vi "Read next.vi"(8 "error in (no error)":errorcluster, 11 "NodeType in":refnum<class "ListNodeVirtual.lvclass">) -> (0 "error out":errorcluster, 2 "next":refnum<data-value>, 3 "NodeType out":refnum<class "ListNodeVirtual.lvclass">)   [LabVIEW 2010, in "ListNodeVirtual.lvclass"]
uses:
  ListNodeVirtual.lvclass
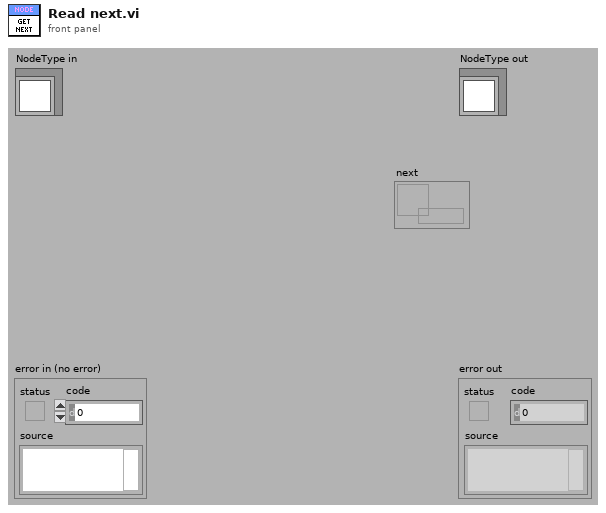
[diagram p1: front panel]
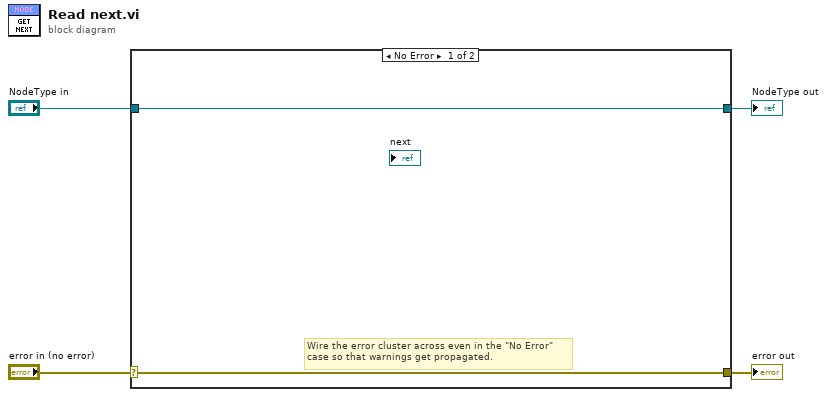
[diagram p0: block diagram]
diagram:
  n1 = case shown="No Error" "error in (no error)" {
    selector: "error in (no error)" -> [w5 w8]
    tunnel: [w5 w8] -> w3
    tunnel: [w6 w7] -> w1
    tunnel: "NodeType in" -> [w6 w7]
    frame No Error {
      # "Wire the error cluster across even in the \"No Error\"\ncase so that warnings get propagated."
    }
    frame Error {
    }
  }
  "error out" <- w3
  "NodeType out" <- w1
